vi "SWLDA_통합버전용.vi"(5 "premove":dbl=0.5, 7 "penter":dbl=0.4, 8 "DIscard Channel Info":i32[](array[numeric]), 9 "ERP_Nontarget":dbl[][](array[numeric]) format="%0.3f", 11 "ERP_Target":dbl[][](array[numeric]) format="%0.3f") -> (2 "in":dbl[](array[numeric]), 3 "LDA_matrix":T1, 6 "WEIGHT":dbl[](array[numeric]))   [LabVIEW 2014]
uses:
  <vilib>/Analysis/Matrix/Datatypes/RealMatrix.ctl
  <vilib>/Analysis/baseanly.llb/Vector x A.vi
  <vilib>/Analysis/Matrix/Numeric/Conversions/Array To Matrix - RA.vi
  <vilib>/Analysis/Matrix/Numeric/Conversions/Array To Matrix - RA2.vi
  <vilib>/Analysis/Matrix/NI_Matrix.lvlib
  <vilib>/Analysis/NI_AALBase.lvlib
panel:
  out "biase":dbl[](array[numeric])
  out "Nontarget_mean":dbl[](array[numeric])
  out "Target_mean":dbl[](array[numeric])
  out "Label":dbl[](array[numeric])
  out "Weight":dbl[](array[numeric])
  # "Target/Non-Target of MATLAB"
  # "var_argin part of MATLAB"
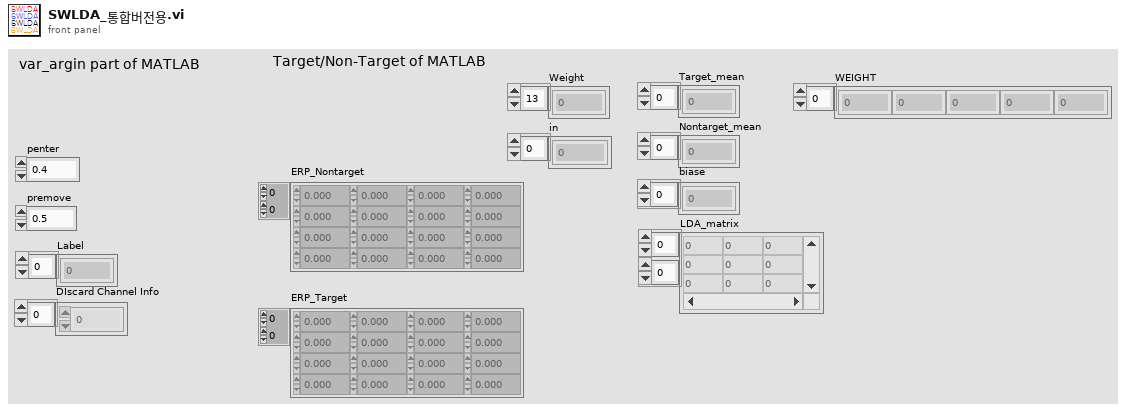
[diagram p1: front panel]
types:
  T1 = typedef "NI_Matrix.lvlib/RealMatrix.ctl" = dbl[][]
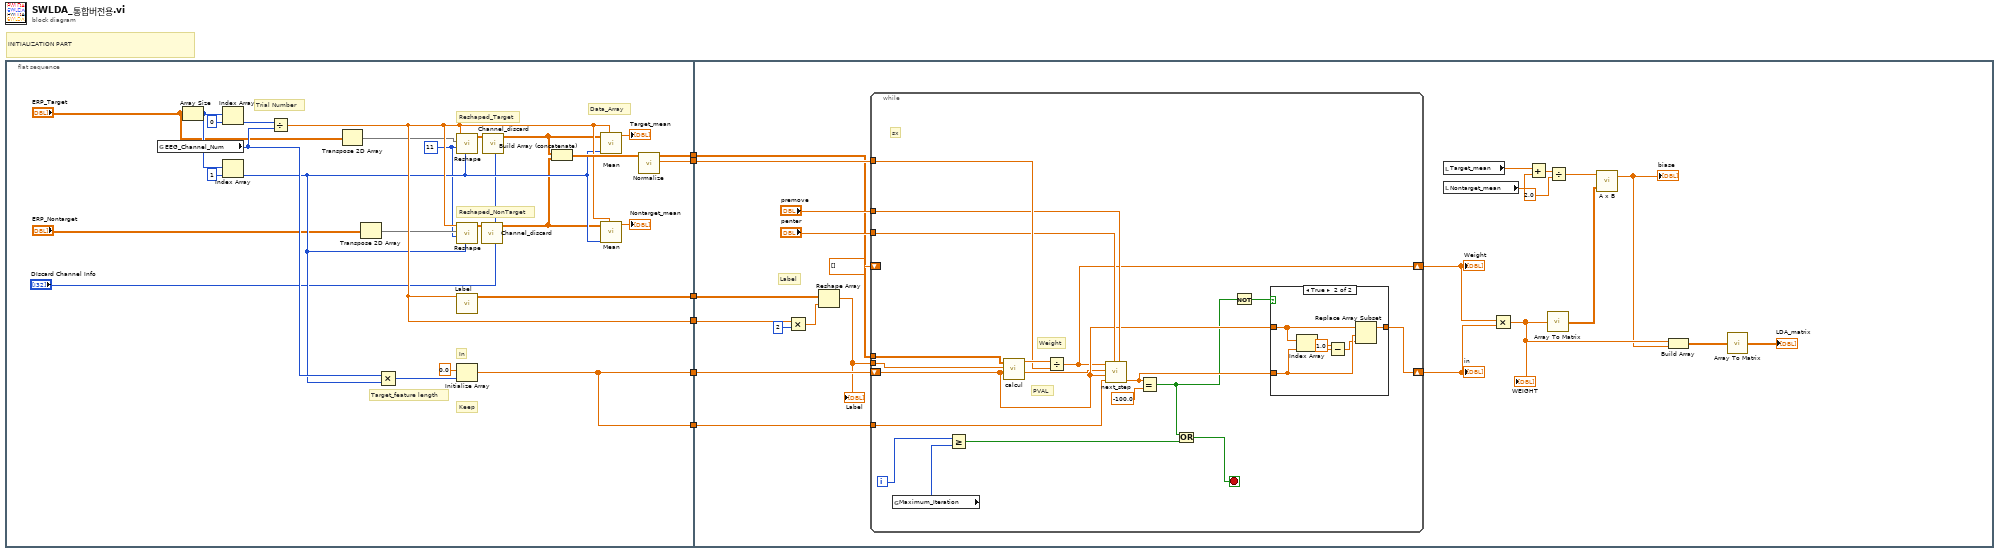
[diagram p0: block diagram]
diagram:
  # "INITIALIZATION PART"
  n1 = flat-sequence {
    tunnel: [w21] -> w6
    tunnel: [w21] -> w5
    tunnel: [w25] -> w4
    tunnel: [w24] -> w3
    tunnel: [w23] -> w2
    tunnel: [w19] -> w1
    tunnel: w6 -> [w55]
    tunnel: w5 -> [w50]
    tunnel: w4 -> [w56]
    tunnel: w3 -> [w46]
    tunnel: w2 -> [w53]
    tunnel: w1 -> [w45]
    frame #0 {
      w8 = 11 ("EEG_Channel_Num")
      # "Keep"
      # "In"
      # "Target_feature length"
      # "Data_Array"
      # "Reshaped_NonTarget"
      # "Reshaped_Target"
      # "Trial Number"
      n2 = global read "Control_Panel_정리.vi" "EEG_Channel_Num"() -> (w28:i32)
      n3 = Array Size(array="ERP_Target") -> (size(s)=w30:i32[])
      n4 = Index Array(array=w30, index=0) -> (element=w29:i32)
      n5 = Index Array(array=w30, index=1) -> (element=w18:i32)
      n6 = Divide(x=w29, y=w28) -> (x/y=w19:dbl)
      n7 = Transpose 2D Array(2D array="ERP_Target") -> (transposed array=w16:dbl[][])
      n8 = Transpose 2D Array(2D array="ERP_Nontarget") -> (transposed array=w15:dbl[][])
      n9 = Multiply(x=w28, y=w18) -> (x*y=w27:i32)
      n10 = call "Reshape.vi"("Numeric"=w18, "EEG_Channel_Num"=w8, "all rows"=w16, "Numeric 2"=w19) -> ("Array"=w14:dbl[][])  [unwired: 7 in]
      n11 = call "Reshape.vi"("Numeric"=w18, "EEG_Channel_Num"=w8, "all rows"=w15, "Numeric 2"=w19) -> ("Array"=w11:dbl[][])  [unwired: 7 in]
      n12 = call "Label.vi"("Numeric"=w19) -> ("Array"=w25:dbl[][])  [unwired: 10 in]
      n13 = Initialize Array(0.0 ("element"), w27) -> (w21:dbl[])
      n14 = call "Channel_discard.vi"("DIscard Channel Info"="DIscard Channel Info", "Array"=w11) -> ("array w/ subset deleted"=w9:dbl[][])  [unwired: 9 in]
      n15 = call "Channel_discard.vi"("DIscard Channel Info"="DIscard Channel Info", "Array"=w14) -> ("array w/ subset deleted"=w10:dbl[][])  [unwired: 9 in]
      n16 = Build Array (concatenate)(w10, w9) -> (w22:dbl[][])
      n17 = call "Mean.vi"("trial_number"=w19, "feature_number"=w18, "Target/NonTarget"=w10) -> ("mean"=→"Target_mean":dbl[])  [unwired: 8 in]
      n18 = call "Mean.vi"("trial_number"=w19, "feature_number"=w18, "Target/NonTarget"=w9) -> ("mean"=→"Nontarget_mean":dbl[])  [unwired: 8 in]
      n19 = call "Normalize.vi"("Data"=w22) -> ("sx"=w23:dbl[], "Data_out"=w24:dbl[][])  [unwired: 8 in, 1 out]
    }
    frame #1 {
      # "Label"
      n20 = Multiply(x=w45, y=2) -> (x*y=w48:dbl)
      n21 = Reshape Array(w56, w48) -> (w54:dbl[])
      "Label" <- w54
      n22 = while {
        shift-right: [w63] -> w37
        shift-left: w55 -> [w64]
        tunnel: w54 -> [w72]
        tunnel: w46 -> [w71]
        tunnel: w53 -> [w69]
        tunnel: "penter" -> [w68]
        tunnel: "premove" -> [w67]
        tunnel: w50 -> [w66]
        shift-right: [w62] -> w38
        shift-left: dbl[] [] -> [_]
        i -> [w75]
        stop <- w73 stop-if-true
        # "sx"
        # "PVAL"
        # "Weight"
        n23 = global read "Control_Panel_정리.vi" "Maximum_Iteration"() -> (w57:i64)
        n24 = Greater Or Equal?(x=w75, y=w57) -> (x >= y?=w74:bool)
        n25 = call "calcul.vi"("In"=w64, "Label (y)"=w72, "Data (allx)"=w71) -> ("PVAL"=w58:dbl[], "B"=w70:dbl[])  [unwired: 7 in]
        n26 = Divide(x=w70, y=w69) -> (x/y=w62:dbl[])
        n27 = call "next_step.vi"("premove"=w67, "penter"=w68, "keep"=w66, "in"=w64, "PVal"=w58, "B"=w62) -> ("swap"=w61:dbl)  [unwired: 4 in, 1 out]
        n28 = Equal?(x=w61, y=-100.0) -> (x = y?=w59:bool)
        n29 = Or(x=w59, y=w74) -> (x .or. y?=w73:bool)
        n30 = Not(x=w59) -> (.not. x?=w60:bool)
        n31 = case shown="True" w60 {
          tunnel: w64 -> [w76 w81]
          tunnel: w61 -> [_ w80]
          tunnel: [w76 w82] -> w63
          frame False {
          }
          frame True {
            n32 = Index Array(array=w81, index=w80) -> (element=w79:dbl)
            n33 = Subtract(x=1.0, y=w79) -> (x-y=w77:dbl)
            n34 = Replace Array Subset(array=w81, new element=w77, index=w80) -> (w82:dbl[])
          }
        }
      }
      "Weight" <- w38
      "in" <- w37
      n35 = local read "Target_mean"() -> (w44:dbl[])
      n36 = local read "Nontarget_mean"() -> (w43:dbl[])
      n37 = Multiply(x=w38, y=w37) -> (x*y=w36:dbl[])
      "WEIGHT" <- w36
      n38 = Add(x=w44, y=w43) -> (x+y=w42:dbl[])
      n39 = call-poly <vilib>:"Array To Matrix.vi"("Real 1D Array"=w36) -> ("Real Matrix (Column Vector)"=w39:T1)
      n40 = Divide(x=w42, y=2.0) -> (x/y=w40:dbl[])
      n41 = call-poly <vilib>:"A x B.vi"("Matrix A"=w39, "Vector V'"=w40) -> ("V' x A"=w35:dbl[])  [unwired: 1 out]
      "biase" <- w35
      n42 = Build Array(w36, w35) -> (w33:dbl[][])
      n43 = call-poly <vilib>:"Array To Matrix.vi"("Real 2D Array"=w33) -> ("Real Matrix"=→"LDA_matrix":T1)
    }
  }
